vi "dataqsdk.vi"() -> ()   [LabVIEW 2019]
panel:
  in  "SampleRate":dbl=1000.0
  in  "DeviceDriver":string="DI320NT.DLL"
  out "Waveform Chart":dbl[][](graph)
  out "Channel 2":dbl(knob) scale=-10.0..10.0
  out "Channel 1":dbl(knob) scale=-10.0..10.0
  in  "DataqSdk":refnum<k7>(container)
  in  "Start/Stop":bool
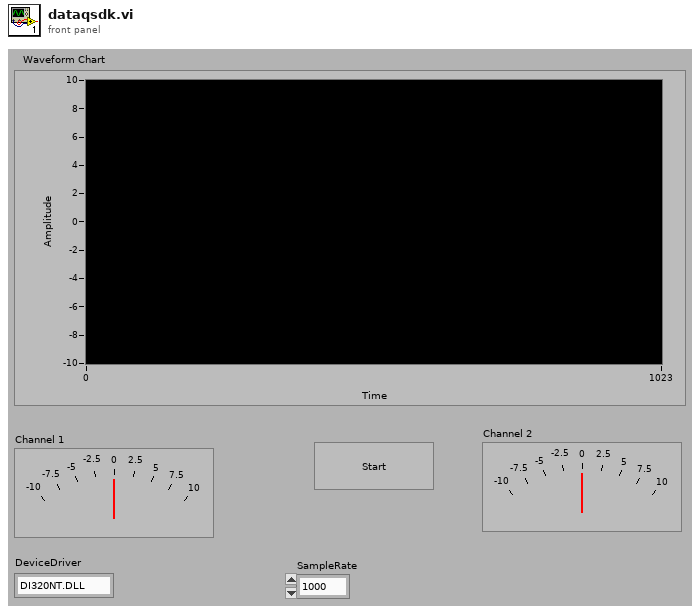
[diagram p1: front panel]
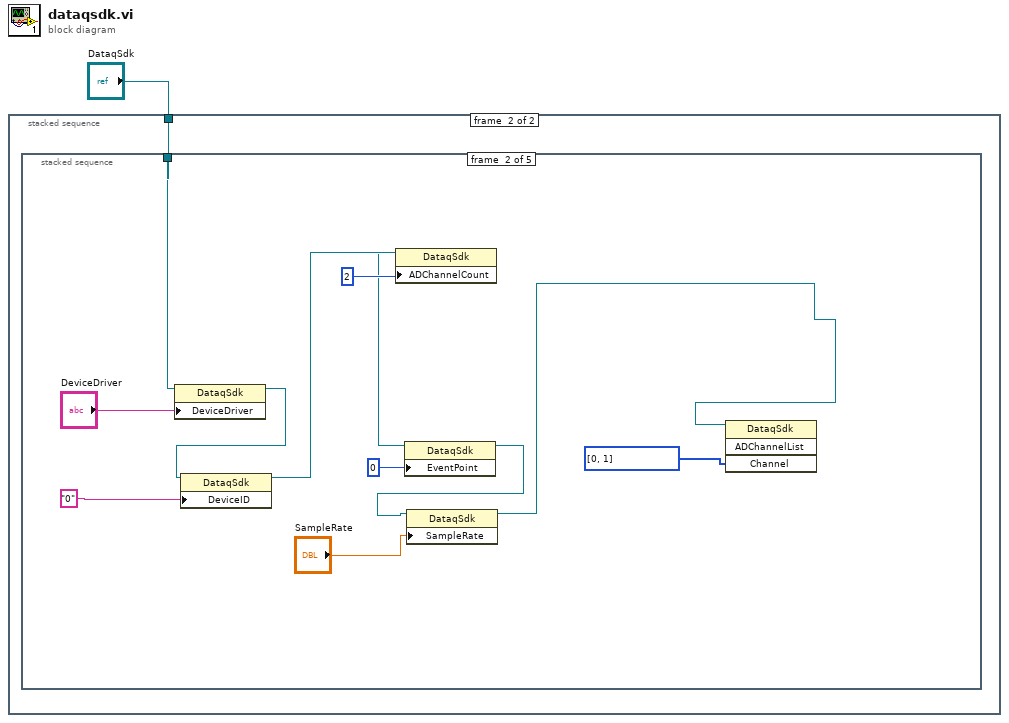
[diagram p0: block diagram]
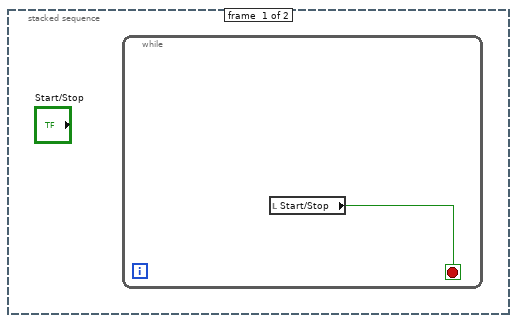
[diagram p2: hidden frame]
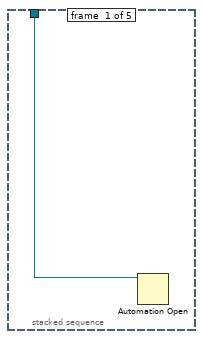
[diagram p3: hidden frame]
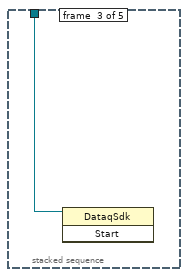
[diagram p4: hidden frame]
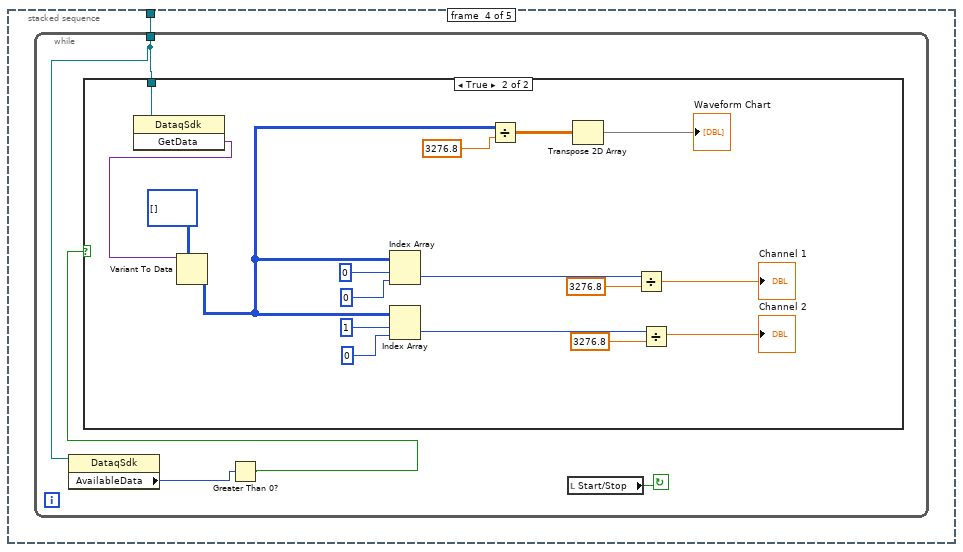
[diagram p5: hidden frame]
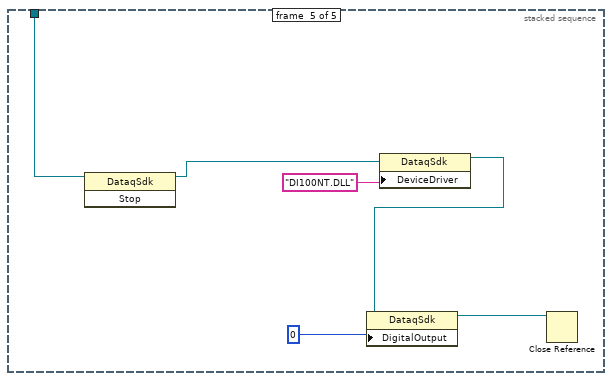
[diagram p7: hidden frame]
diagram:
  n1 = stacked-sequence {
    tunnel: "DataqSdk" -> [_ w3]
    frame #0 {
      n2 = while {
        stop <- w2 stop-if-true
        n3 = local read "Start/Stop"() -> (w2:bool)
      }
    }
    frame #1 {
      n4 = stacked-sequence {
        tunnel: w3 -> [w4 w11 w17 w18 w45]
        frame #0 {
          n5 = Automation Open(Automation Refnum=w4) -> ()  [unwired: 3 in, 2 out]
        }
        frame #1 {
          n6 = property class="DataqSdk"(reference=w11, "DeviceDriver"="DeviceDriver") -> (reference out=w10:refnum<k7>)  [unwired: 1 in, 1 out]
          n7 = property class="DataqSdk"(reference=w10, "DeviceID"="0") -> (reference out=w9:refnum<k7>)  [unwired: 1 in, 1 out]
          n8 = property class="DataqSdk"(reference=w9, "ADChannelCount"=2) -> (reference out=w8:refnum<k7>)  [unwired: 1 in, 1 out]
          n9 = property class="DataqSdk"(reference=w8, "EventPoint"=0) -> (reference out=w7:refnum<k7>)  [unwired: 1 in, 1 out]
          n10 = property class="DataqSdk"(reference=w7, "SampleRate"="SampleRate") -> (reference out=w5:refnum<k7>)  [unwired: 1 in, 1 out]
          n11 = invoke class="DataqSdk" method="ADChannelList"(reference=w5, "Channel"=i32[] [0, 1] ("Array")) -> ()  [unwired: 2 in, 4 out]
        }
        frame #2 {
          n12 = invoke class="DataqSdk" method="Start"(reference=w17) -> ()  [unwired: 2 in, 3 out]
        }
        frame #3 {
          n13 = while {
            tunnel: w18 -> [w21]
            stop <- w22 continue-if-true
            n14 = property class="DataqSdk"(reference=w21) -> ("AvailableData"=w20:i32)  [unwired: 1 in, 2 out]
            n15 = Greater Than 0?(x=w20) -> (x > 0?=w19:bool)
            n16 = case shown="True" w19 {
              tunnel: w21 -> [_ w39]
              frame False {
              }
              frame True {
                n17 = invoke class="DataqSdk" method="GetData"(reference=w39) -> ("GetData"=w35:variant)  [unwired: 2 in, 2 out]
                n18 = Variant To Data(type=i16[][] [], Variant=w35) -> (data=w25:i16[][])  [unwired: 1 in, 1 out]
                n19 = Index Array(array=w25, index (row)=0, index (col)=0) -> (element=w24:i16)
                n20 = Index Array(array=w25, index (row)=1, index (col)=0) -> (element=w23:i16)
                n21 = Divide(x=w25, y=3276.8) -> (x/y=w29:dbl[][])
                n22 = Transpose 2D Array(2D array=w29) -> (transposed array=→"Waveform Chart":dbl[][])
                n23 = Divide(x=w24, y=3276.8) -> (x/y=→"Channel 1":dbl)
                n24 = Divide(x=w23, y=3276.8) -> (x/y=→"Channel 2":dbl)
              }
            }
            n25 = local read "Start/Stop"() -> (w22:bool)
          }
        }
        frame #4 {
          n26 = invoke class="DataqSdk" method="Stop"(reference=w45) -> (reference out=w44:refnum<k7>)  [unwired: 2 in, 2 out]
          n27 = property class="DataqSdk"(reference=w44, "DeviceDriver"="DI100NT.DLL") -> (reference out=w43:refnum<k7>)  [unwired: 1 in, 1 out]
          n28 = property class="DataqSdk"(reference=w43, "DigitalOutput"=0) -> (reference out=w42:refnum<k7>)  [unwired: 1 in, 1 out]
          n29 = Close Reference(reference=w42) -> ()  [unwired: 1 in, 1 out]
        }
      }
    }
  }
